vi "Load App.vi"(8 "error in (no error)":cluster{"状态":bool, "代码":i32, "源":string} caption="错误输入（无错误）", 11 "状态通知器":refnum<notifier>) -> (0 "error out":cluster{"状态":bool, "代码":i32, "源":string} caption="错误输出")   [LabVIEW 2013, in "Air Cooler Application.lvlib" / "Air Cooler Application.lvclass"]
doc: "执行加载应用程序时的必要操作。输入通知器用于将文本发送至初始屏幕。这些文本向用户显示加载进程当前的状态。"
uses:
  Air Cooler Application.lvclass
  <vilib>/ActorFramework/Message Queue/Message Queue.lvclass/Message Queue.ctl
  <vilib>/ActorFramework/Actor/Actor.lvclass
  <vilib>/ActorFramework/Message Queue/Message Queue.lvclass
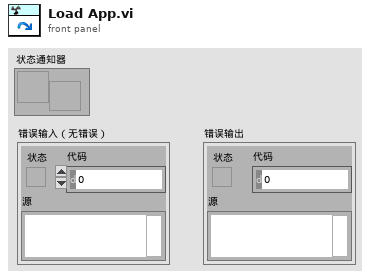
[diagram p1: front panel]
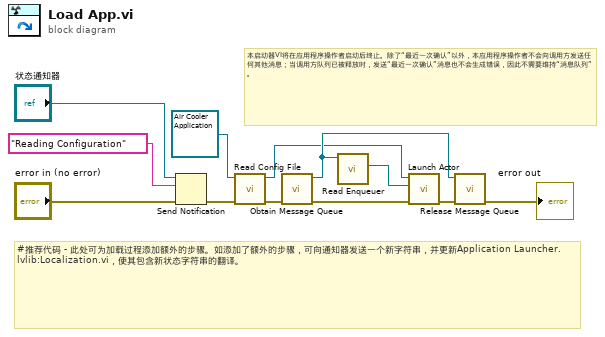
[diagram p0: block diagram]
diagram:
  # "本启动器VI将在应用程序操作者启动后终止。除了“最近一次确认”以外，本应用程序操作者不会向调用方发送任何其他消息；当调用方队列已被释放时，发送“最近一次确认”消息也不会生成错误，因此不需要维持“消息队列”。"
  # "#推荐代码 - 此处可为加载过程添加额外的步骤。如添加了额外的步骤，可向通知器发送一个新字符串，并更新Application Launcher.lvlib:Localization.vi，使其包含新状态字符串的翻译。"
  n1 = Send Notification(notification="Reading Configuration", notifier="状态通知器", error in (no error)="error in (no error)") -> (error out=w8:errorcluster)  [unwired: 1 out]
  n2 = call-dynamic "Read Config File.vi"("error in (no error)"=w8, "气冷系统应用程序输入"=refnum<class "Air Cooler Application.lvclass"> refnum ("My Application.lvclass")) -> ("error out"=w4:cluster{"状态":bool, "代码":i32, "源":string}, "气冷系统应用程序输出"=w1:refnum<class "Air Cooler Application.lvclass">)  [unwired: 8 in]
  n3 = call <vilib>:"Obtain Message Queue.vi"("error in (no error)"=w4) -> ("error out"=w3:errorcluster, "Message Queue"=w2:refnum<class "Message Queue.lvclass">)  [unwired: 9 in]
  n4 = call <vilib>:"Read Enqueuer.vi"("Message Queue"=w2) -> ("Message Enqueuer"=w7:refnum<class "Message Enqueuer.lvclass">)  [unwired: 10 in]
  n5 = call <vilib>:"Launch Actor.vi"("error in (no error)"=w3, "Actor-to-Caller Enqueuer"=w7, "Actor"=w1) -> ("error out"=w6:errorcluster)  [unwired: 7 in, 1 out]
  n6 = call <vilib>:"Release Message Queue.vi"("error in (no error)"=w6, "Message Queue"=w2) -> ("error out"=→"error out":errorcluster)  [unwired: 8 in, 1 out]
